vi "get_notification_from_queue.vi"(0 "Error in":errorcluster, 1 "Queue in":refnum<queue>) -> (2 "Error out":errorcluster, 3 "Should act":bool, 4 "Queue out":refnum<queue>)   [LabVIEW 2010]
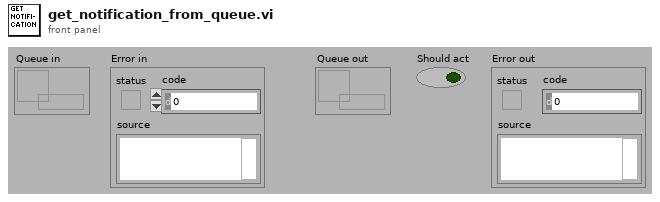
[diagram p1: front panel]
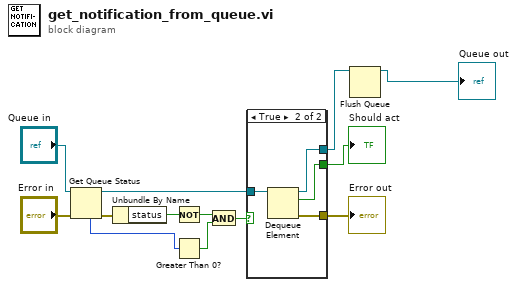
[diagram p0: block diagram]
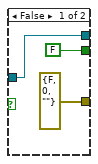
[diagram p2: hidden frame]
diagram:
  n1 = Get Queue Status(queue="Queue in", error in (no error)="Error in") -> (queue out=w9:refnum<queue>, error out=w5:errorcluster, # elements in queue=w4:i32)  [unwired: 1 in, 5 out]
  n2 = Unbundle By Name(w5) -> ("status"=w6:bool)
  n3 = Not(x=w6) -> (.not. x?=w7:bool)
  n4 = Greater Than 0?(x=w4) -> (x > 0?=w8:bool)
  n5 = And(x=w7, y=w8) -> (x .and. y?=w10:bool)
  n6 = case shown="True" w10 {
    tunnel: w9 -> [w16 w20]
    tunnel: [w16 w19] -> w2
    tunnel: [FALSE w18] -> w11
    tunnel: [errorcluster {"status"=FALSE, "code"=0, "source"=""} ("error out") w17] -> w12
    frame False {
    }
    frame True {
      n7 = Dequeue Element(queue=w20) -> (queue out=w19:refnum<queue>, element=w18:bool, error out=w17:errorcluster)  [unwired: 2 in, 1 out]
    }
  }
  "Error out" <- w12
  "Should act" <- w11
  n8 = Flush Queue(queue=w2) -> (queue out=→"Queue out":refnum<queue>)  [unwired: 1 in, 2 out]
